vi "GetAnalogInput.vi"(4 "error in (no error)":errorcluster, 6 "analog input number":u16=1, 7 "axis in":cluster{"keyHandle":u32, "nodeId":u16}={"keyHandle"=0, "nodeId"=1}) -> (0 "error out":errorcluster, 2 "analog input value":u16, 3 "axis out":cluster{"keyHandle":u32, "nodeId":u16}={"keyHandle"=0, "nodeId"=1})   [LabVIEW 2017, in "maxonEPOS.lvlib"]
doc: "<B>GetAnalogInput</B> reads the analog value from an input from the device."
uses:
  Examples/maxonEPOS.lvlib
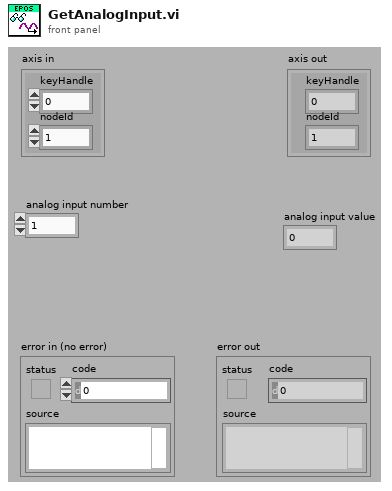
[diagram p1: front panel]
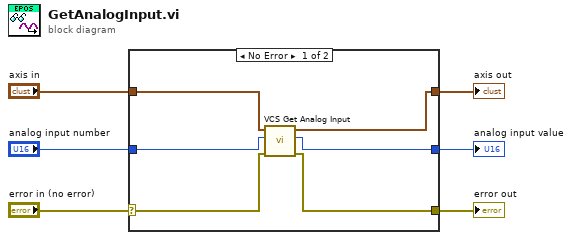
[diagram p0: block diagram]
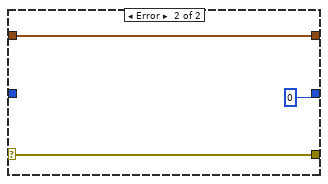
[diagram p2: hidden frame]
diagram:
  n1 = case shown="No Error" "error in (no error)" {
    selector: "error in (no error)" -> [w8 w15]
    tunnel: [w7 w15] -> w5
    tunnel: [w10 w14] -> w4
    tunnel: "axis in" -> [w9 w14]
    tunnel: "analog input number" -> [w12 _]
    tunnel: [w11 u16 0 ("analogInput")] -> w1
    frame No Error {
      n2 = call "VCS Get Analog Input.vi"("error in (no error)"=w8, "number"=w12, "axis in"=w9) -> ("error out"=w7:errorcluster, "analogInput"=w11:u16, "axis out"=w10:cluster{"keyHandle":u32, "nodeId":u16})  [unwired: 6 in]
    }
    frame Error {
    }
  }
  "error out" <- w5
  "axis out" <- w4
  "analog input value" <- w1
